vi "Temperature Limit.vi"() -> ()   [LabVIEW 2015]
doc: "This VI simulates the acquisition of temperature, graphs the temperature, and notifies the user if the temperature is over the limit."
panel:
  in  "Tool Bar:Visible":bool
  in  "Start":bool
  in  "Delta t (ms)":i32(slide)=400 scale=50.0..500.0
  in  "Stop":bool
  in  "High Limit":dbl=28.0 format="%.2f"
  out "Temperature":cluster{"Temperature":dbl, "High Limit":dbl}(graph)={"Temperature"=85.88749999999999, "High Limit"=80.0}
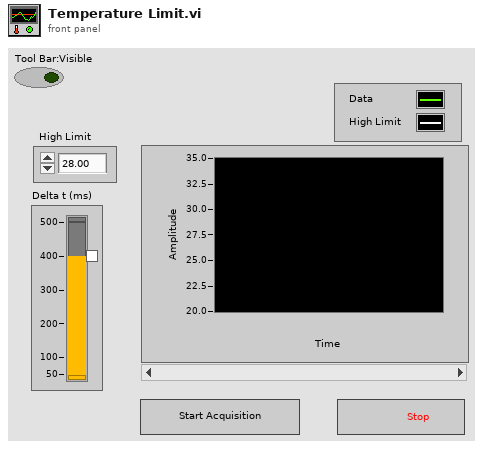
[diagram p1: front panel]
types:
  T1 = enum16{"Always On", "Always Off", "Off While Running"}
  T2 = cluster{"Temperature Value":dbl, "High Limit":dbl}
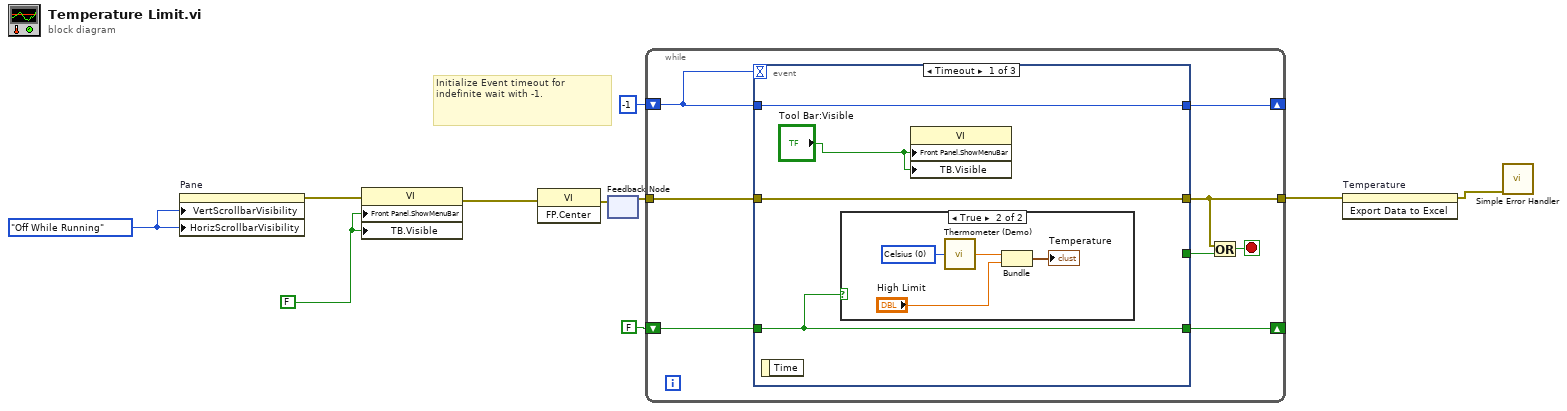
[diagram p0: block diagram]
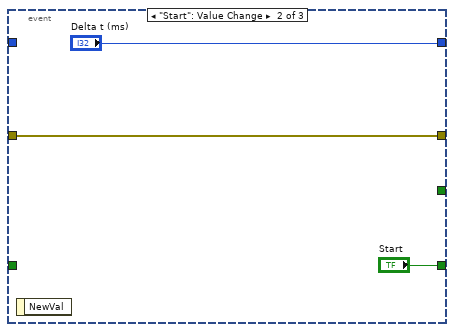
[diagram p3: hidden frame]
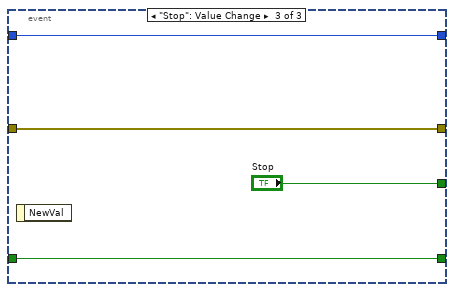
[diagram p4: hidden frame]
diagram:
  w3 = FALSE ("Tool Bar:Visible")
  w8 = T1."Off While Running" ("Horizontal Scrollbar Visibility")
  # "Initialize Event timeout for indefinite wait with -1."
  n1 = property on="Pane" class="Pane"("VertScrollbarVisibility"=w8, "HorizScrollbarVisibility"=w8) -> (error out=w7:errorcluster)  [unwired: 2 in, 1 out]
  n2 = property class="VI"(error in=w7, "Front Panel.ShowMenuBar"=w3, "TB.Visible"=w3) -> (error out=w6:errorcluster)  [unwired: 1 in, 1 out]
  n3 = invoke class="VI" method="FP.Center"(error in=w6) -> (error out=w5:errorcluster)  [unwired: 2 in, 2 out]
  n4 = feedback-in #1(w5) -> ()
  n5 = feedback #1() -> (w4:errorcluster)  [unwired: 1 in]
  n6 = while {
    tunnel: w4 -> [w18]
    tunnel: [w16] -> w2
    shift-right: [w14] -> _
    shift-left: FALSE ("Start") -> [w13]
    shift-right: [w12] -> _
    shift-left: -1 ("Delta t (ms)") -> [w11]
    stop <- w17 stop-if-true
    n7 = event shown="[0] Timeout" {
      selector: _ -> [_ _ _]
      dyn-events: _ -> [_ _ _]
      timeout: w11 -> [_ _ _]
      tunnel: [_ _ "Stop"] -> w15
      tunnel: w18 -> [w22 w27 w32]
      tunnel: [w22 w27 w32] -> w16
      tunnel: [w20 "Start" w31] -> w14
      tunnel: w13 -> [w20 _ w31]
      tunnel: [w21 "Delta t (ms)" w30] -> w12
      tunnel: w11 -> [w21 _ w30]
      event Timeout {
        n8 = event-data() -> ()  [unwired: 1 in, 1 out]
        n9 = case shown="True" w20 {
          frame False {
          }
          frame True {
            w23 = u16 0 items=["Celsius", "Fahrenheit"] ("Units (0: Celsius)")
            n10 = call "Thermometer (Demo).vi"("Units (0: Celsius)"=w23) -> ("Temperature Value"=w24:dbl)
            n11 = Bundle("Temperature Value"=w24, "High Limit"="High Limit") -> (→"Temperature":T2)  [unwired: 1 in]
          }
        }
        n12 = property class="VI"("Front Panel.ShowMenuBar"="Tool Bar:Visible", "TB.Visible"="Tool Bar:Visible") -> ()  [unwired: 2 in, 2 out]
      }
      event "Start": Value Change {
        n13 = event-data() -> ()  [unwired: 1 in, 1 out]
      }
      event "Stop": Value Change {
        n14 = event-data() -> ()  [unwired: 1 in, 1 out]
      }
    }
    n15 = Or(x=w16, y=w15) -> (x .or. y?=w17:bool)
  }
  n16 = invoke on="Temperature" class="WFChart (strict)" method="Export Data to Excel"(error in=w2) -> (error out=w1:errorcluster)  [unwired: 2 in, 2 out]
  n17 = call <vilib>:"Simple Error Handler.vi"("error in (no error)"=w1) -> ()  [unwired: 4 in, 5 out]
